vi "Voltage_Check.vi"(0 "channel1":dbl, 1 "limitmin":dbl, 2 "channel2":dbl, 3 "channel3":dbl, 4 "limitmax":dbl, 5 "channel4":dbl, 6 "error in (no error) 2":errorcluster) -> (7 "state":bool, 8 "error out 2":errorcluster)   [LabVIEW 2015]
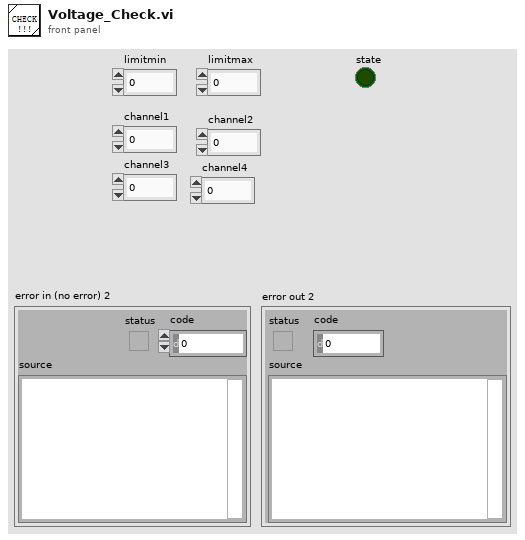
[diagram p1: front panel]
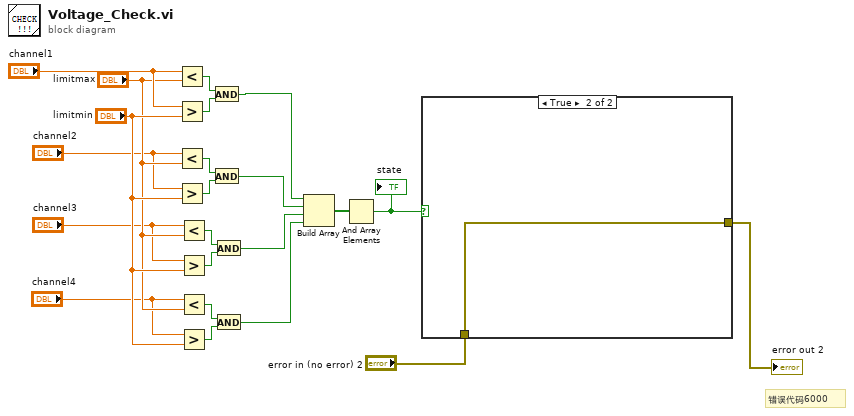
[diagram p0: block diagram]
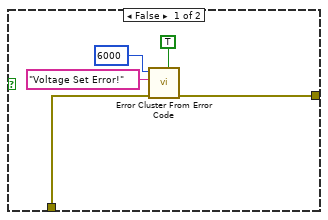
[diagram p2: hidden frame]
diagram:
  # "错误代码6000"
  n1 = Less?(x="channel1", y="limitmax") -> (x < y?=w21:bool)
  n2 = Greater?(x="channel1", y="limitmin") -> (0:w22:bool)
  n3 = Less?(x="channel2", y="limitmax") -> (x < y?=w19:bool)
  n4 = Greater?(x="channel2", y="limitmin") -> (0:w20:bool)
  n5 = Less?(x="channel3", y="limitmax") -> (x < y?=w17:bool)
  n6 = Greater?(x="channel3", y="limitmin") -> (0:w18:bool)
  n7 = Less?(x="channel4", y="limitmax") -> (x < y?=w15:bool)
  n8 = Greater?(x="channel4", y="limitmin") -> (0:w16:bool)
  n9 = And(x=w21, y=w22) -> (x .and. y?=w8:bool)
  n10 = And(x=w19, y=w20) -> (x .and. y?=w7:bool)
  n11 = And(x=w17, y=w18) -> (x .and. y?=w6:bool)
  n12 = And(x=w15, y=w16) -> (x .and. y?=w5:bool)
  n13 = Build Array(w8, w7, w6, w5) -> (w4:bool[])
  n14 = And Array Elements(Boolean array=w4) -> (logical AND=w3:bool)
  "state" <- w3
  n15 = case shown="True" w3 {
    tunnel: "error in (no error) 2" -> [w27 w28]
    tunnel: [w26 w28] -> w1
    frame False {
      n16 = call <vilib>:"Error Cluster From Error Code.vi"("is warning? (False)"=TRUE, "error in (no error)"=w27, "error message (\"\")"="Voltage Set Error!" ("error message (\"\")"), "error code (0)"=6000) -> ("error out"=w26:errorcluster)  [unwired: 5 in]
    }
    frame True {
    }
  }
  "error out 2" <- w1
